vi "Clean_Barrier.vi"(4 "Replaced With (Y)":i32[](array[numeric]), 5 "Replaced With (X)":i32[](array[numeric]), 6 "Removed and Ignored (Y)":i32[](array[numeric]), 7 "Removed and Ignored (X)":i32[](array[numeric]), 11 "Barriers":T1[](array[typedef])) -> (3 "Barriers 2":T1[](array[typedef]))   [LabVIEW 2016]
uses:
  Controls/Parse-(X,Y).ctl
  Controls/TileColor.ctl
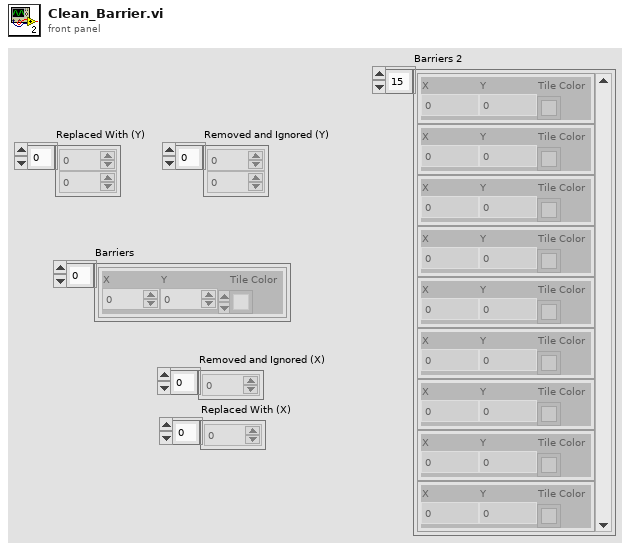
[diagram p1: front panel]
types:
  T1 = typedef "Parse-(X,Y).ctl" = cluster{"X":i32, "Y":i32, "Tile Color":T2}
  T2 = typedef "TileColor.ctl" = u16
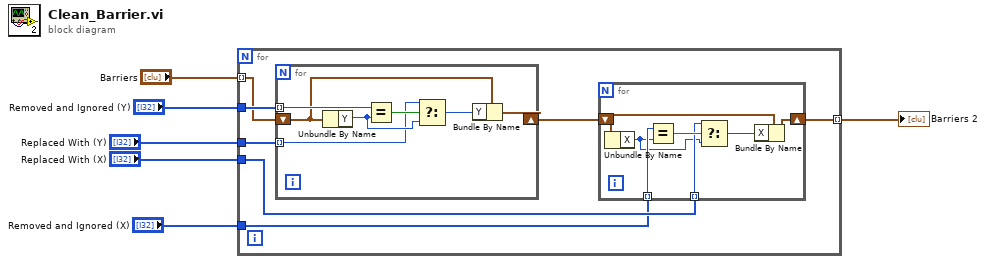
[diagram p0: block diagram]
diagram:
  n1 = for {
    tunnel: "Barriers" -> [w12] mode=indexing
    tunnel: "Removed and Ignored (Y)" -> [w13]
    tunnel: "Replaced With (Y)" -> [w11]
    tunnel: [w9] -> w3 mode=indexing
    tunnel: "Removed and Ignored (X)" -> [w7]
    tunnel: "Replaced With (X)" -> [w8]
    n2 = for {
      tunnel: w13 -> [w27] mode=indexing
      tunnel: w11 -> [w22] mode=indexing
      shift-right: [w21] -> w10
      shift-left: w12 -> [w25]
      n3 = Unbundle By Name(w25) -> ("Y"=w23:i32)
      n4 = Equal?(x=w27, y=w23) -> (x = y?=w26:bool)
      n5 = Select(t=w22, s=w26, f=w23) -> (s? t:f=w24:i32)
      n6 = Bundle By Name(cluster=w25, "Y"=w24) -> (w21:T1)
    }
    n7 = for {
      shift-right: [w16] -> w9
      shift-left: w10 -> [w17]
      tunnel: w8 -> [w18] mode=indexing
      tunnel: w7 -> [w15] mode=indexing
      n8 = Unbundle By Name(w17) -> ("X"=w14:i32)
      n9 = Equal?(x=w15, y=w14) -> (x = y?=w19:bool)
      n10 = Select(t=w18, s=w19, f=w14) -> (s? t:f=w20:i32)
      n11 = Bundle By Name(cluster=w17, "X"=w20) -> (w16:T1)
    }
  }
  "Barriers 2" <- w3
